vi "Zero Terminated Byte Array to String.vi"(4 "byte array":u8[](array[numeric]) format="%.0x") -> (1 "string":string)   [LabVIEW 2014, in "PICam.lvlib"]
uses:
  PICam.lvlib
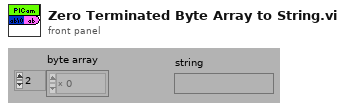
[diagram p1: front panel]
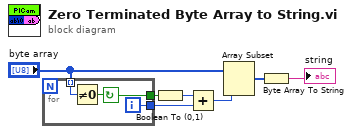
[diagram p0: block diagram]
diagram:
  n1 = for {
    tunnel: "byte array" -> [w10] mode=indexing
    tunnel: [w9] -> w4
    tunnel: [w8] -> w1
    i -> [w9]
    stop <- w8 continue-if-true
    n2 = Not Equal To 0?(x=w10) -> (x != 0?=w8:bool)
  }
  n3 = Boolean To (0,1)(Boolean=w1) -> (0, 1=w2:i16)
  n4 = Add(x=w2, y=w4) -> (x+y=w3:i32)
  n5 = Array Subset(array="byte array", length=w3) -> (w6:u8[])  [unwired: 1 in]
  n6 = Byte Array To String(unsigned byte array=w6) -> (string=→"string":string)
